vi "Write Ctrl_.vi"(8 "error in (no error)":errorcluster, 10 "Ctrl?":bool, 11 "Keyboard Macro in":refnum<class "Keyboard Macro.lvclass">) -> (0 "error out":errorcluster, 3 "Keyboard Macro out":refnum<class "Keyboard Macro.lvclass">)   [LabVIEW 2020, in "MacroAssert.lvlib" / "Keyboard Macro.lvclass"]
uses:
  Keyboard Macro.lvclass
  Keyboard Macro.lvclass/Keyboard Macro.ctl
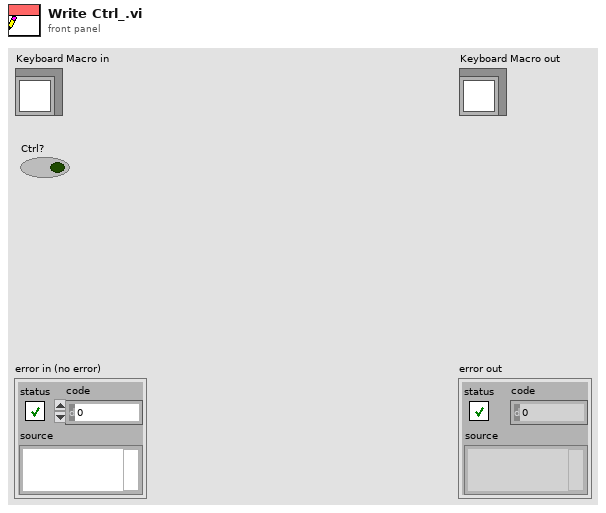
[diagram p1: front panel]
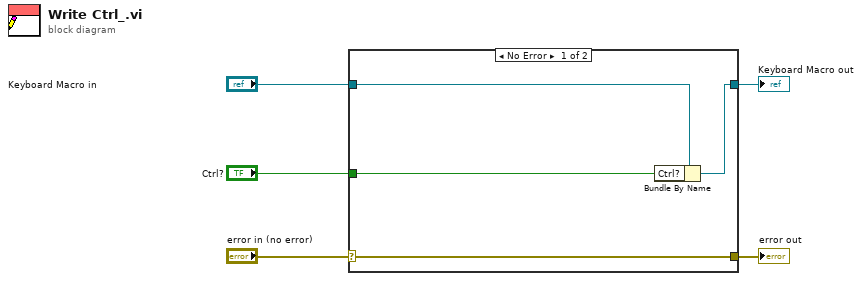
[diagram p0: block diagram]
diagram:
  n1 = case shown="No Error" "error in (no error)" {
    selector: "error in (no error)" -> [w9 w10]
    tunnel: [w9 w10] -> w4
    tunnel: [w7 w11] -> w2
    tunnel: "Keyboard Macro in" -> [w8 w11]
    tunnel: "Ctrl?" -> [w6 _]
    frame No Error {
      n2 = Bundle By Name(cluster=w8, "Ctrl?"=w6) -> (w7:refnum<class "Keyboard Macro.lvclass">)
    }
    frame Error {
    }
  }
  "error out" <- w4
  "Keyboard Macro out" <- w2
